vi "Clean Up.vi"(8 "error in (no error)":errorcluster, 11 "PXI in":refnum<class "PXI.lvclass">) -> (0 "error out":errorcluster, 3 "PXI out":refnum<class "PXI.lvclass">)   [LabVIEW 2013, in "PXI.lvclass"]
uses:
  PXI.lvclass
  PXI.lvclass/PXI.ctl
  <resource>/objmgr/daqmx.rc
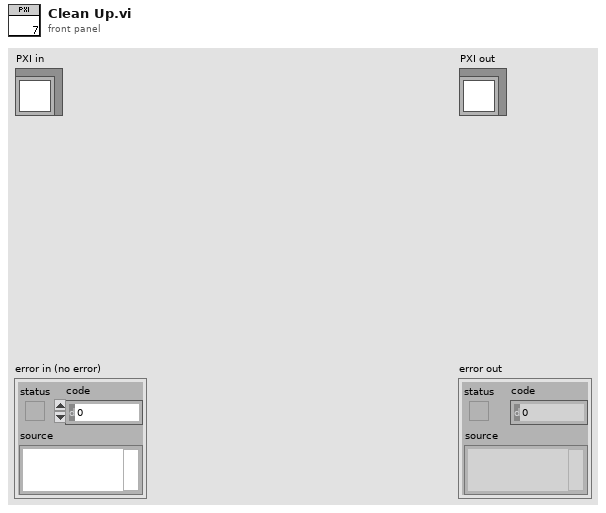
[diagram p1: front panel]
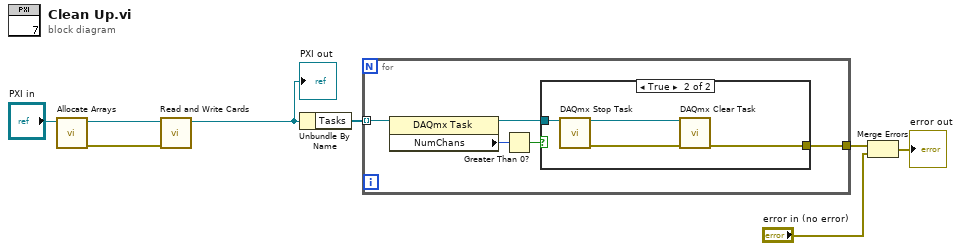
[diagram p0: block diagram]
diagram:
  n1 = call "Allocate Arrays.vi"("PXI in"="PXI in") -> ("error out"=w4:errorcluster, "PXI out"=w7:refnum<class "PXI.lvclass">)  [unwired: 9 in]
  n2 = call "Read and Write Cards.vi"("error in (no error)"=w4, "PXI in"=w7) -> ("PXI out"=w5:refnum<class "PXI.lvclass">)  [unwired: 8 in, 1 out]
  "PXI out" <- w5
  n3 = Unbundle By Name(w5) -> ("Tasks"=w8:refnum<k21>[])
  n4 = for {
    tunnel: w8 -> [w9] mode=indexing
    tunnel: [w10] -> w2
    n5 = property class="DAQmx Task"(reference=w9) -> (reference out=w11:refnum<k21>, "NumChans"=w13:u32)  [unwired: 1 in, 1 out]
    n6 = Greater Than 0?(x=w13) -> (x > 0?=w12:bool)
    n7 = case shown="True" w12 {
      tunnel: w11 -> [_ w15]
      tunnel: [_ w14] -> w10
      frame False {
      }
      frame True {
        n8 = call <vilib>:"DAQmx Stop Task.vi"("task/channels in"=w15) -> ("task out"=w17:refnum<k21>, "error out"=w16:errorcluster)  [unwired: 13 in]
        n9 = call <vilib>:"DAQmx Clear Task.vi"("task in"=w17, "error in"=w16) -> ("error out"=w14:errorcluster)  [unwired: 13 in]
      }
    }
  }
  n10 = Merge Errors(w2, "error in (no error)") -> (→"error out":errorcluster)
